vi "Pelletron_update.vi"(8 "Cluster":T1, 11 "AccelNET.lvlib:PelletronStatus.lvclass":refnum<class "PelletronStatus.lvclass">) -> (3 "AccelNET.lvlib:PelletronStatus.lvclass 2":refnum<class "PelletronStatus.lvclass">)   [LabVIEW 2012, in "AccelNET.lvlib" / "PelletronStatus.lvclass"]
uses:
  PelletronStatus.lvclass
  interface/Pelletron.ctl
  PelletronStatus.lvclass/PelletronStatus.ctl
  interface/Interface.lvlib
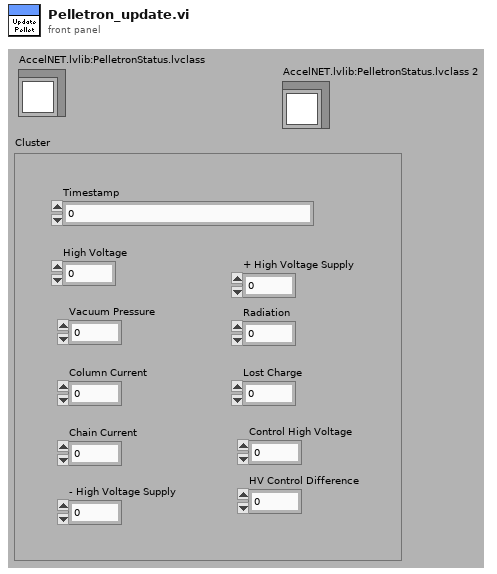
[diagram p1: front panel]
types:
  T1 = typedef "Interface.lvlib/Pelletron.ctl" = cluster{"Timestamp":u64, "High Voltage":sgl, "Vacuum Pressure":sgl, "Column Current":sgl, "Chain Current":sgl, "- High Voltage Supply":dbl, "+ High Voltage Supply":dbl, "Radiation":dbl, "Lost Charge":dbl, "Control High Voltage":dbl, "HV Control Difference":dbl}
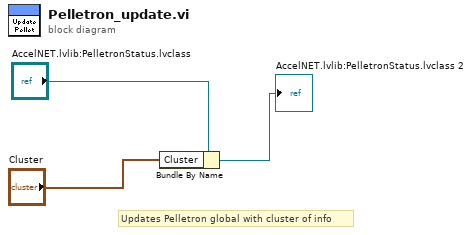
[diagram p0: block diagram]
diagram:
  # "Updates Pelletron global with cluster of info"
  n1 = Bundle By Name(cluster="AccelNET.lvlib:PelletronStatus.lvclass", "Cluster"="Cluster") -> (→"AccelNET.lvlib:PelletronStatus.lvclass 2":refnum<class "PelletronStatus.lvclass">)
